vi "振动NVH.vi"() -> ()   [LabVIEW 2019]
panel:
  out "振动NHV-FFT":cluster{"f0":dbl, "df":dbl, "magnitude":dbl[]}[](graph)
  out "振动NVH-Order":cluster{"f0":dbl, "df":dbl, "magnitude":dbl[]}[](graph)
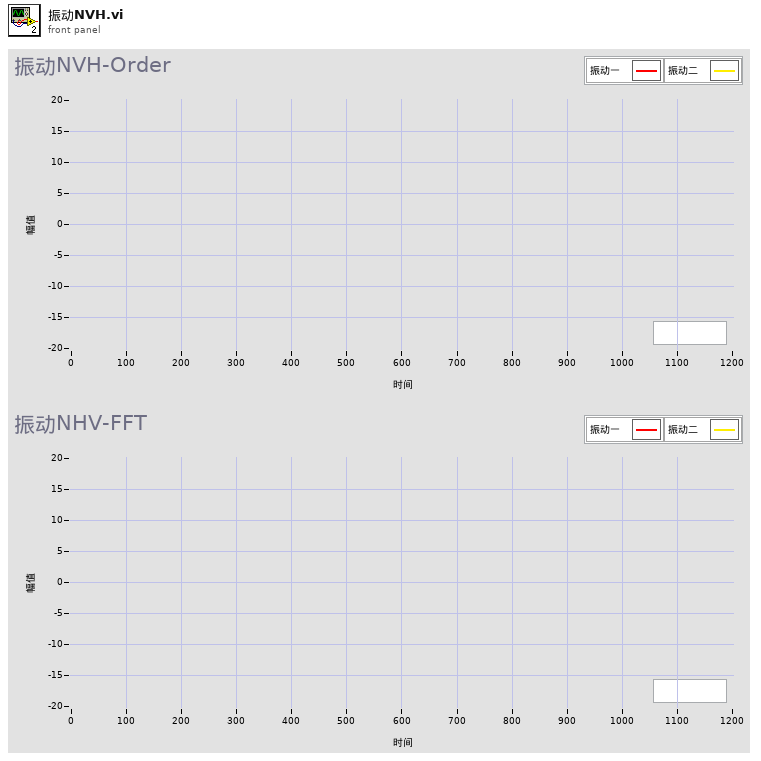
[diagram p1: front panel]
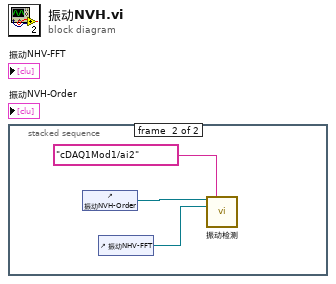
[diagram p0: block diagram]
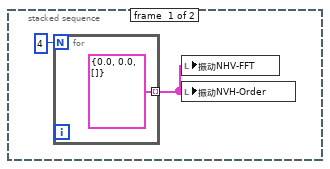
[diagram p2: hidden frame]
diagram:
  n1 = stacked-sequence {
    frame #0 {
      n2 = for {
        N: 4 -> [_]
        tunnel: [cluster{"f0":dbl, "df":dbl, "magnitude":dbl[]} {"f0"=0.0, "df"=0.0, "magnitude"=[]} ("power spectrum [dB EU]")] -> w1 mode=indexing
      }
      n3 = local write "振动NHV-FFT"(w1) -> ()
      n4 = local write "振动NVH-Order"(w1) -> ()
    }
    frame #1 {
      n5 = control-ref of="振动NVH-Order"() -> (w6:refnum<vi>)
      n6 = control-ref of="振动NHV-FFT"() -> (w5:refnum<vi>)
      n7 = call "振动检测.vi"("振动一"=w6, "通道输入"=tag "cDAQ1Mod1/ai2" ("DAQmx物理通道"), "振动二"=w5) -> ()  [unwired: 11 in, 2 out]
    }
  }
